vi "Set Double.vi"(8 "error in":errorcluster, 9 "value":dbl, 10 "variable name":string, 11 "GOLPI ref. in":T1={"pipe handle"={"lv_proc.dll file path"=path "", "process instance handle"=[]}, "fast read timeout [ms]"=500, "fast read settle time [ms]"=10, "fast read to multiple [ms]"=1, "max elements per input line"=100}) -> (0 "error out":errorcluster, 3 "GOLPI ref. out":T1={"pipe handle"={"lv_proc.dll file path"=path "", "process instance handle"=[]}, "fast read timeout [ms]"=500, "fast read settle time [ms]"=10, "fast read to multiple [ms]"=1, "max elements per input line"=100})   [LabVIEW 2013, in "GOLPI library.lvlib"]
uses:
  GOLPI library.lvlib
  Type Definitions/GOLPI reference Type Def.ctl
  LV Process.lvlibp/Pipe Handle.ctl
  LV Process.lvlibp
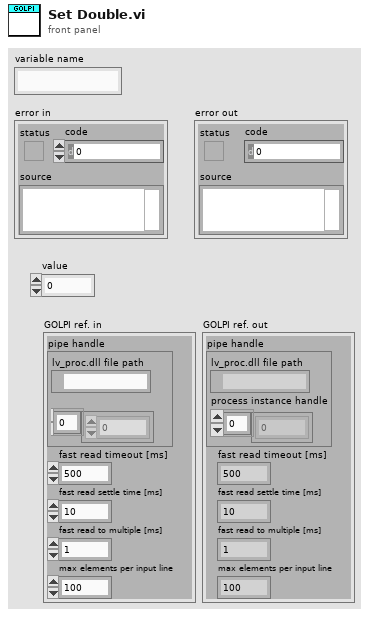
[diagram p1: front panel]
types:
  T1 = typedef "GOLPI library.lvlib/GOLPI reference Type Def.ctl" = cluster{"pipe handle":T2, "fast read timeout [ms]":u32, "fast read settle time [ms]":u32, "fast read to multiple [ms]":u32, "max elements per input line":u32}
  T2 = typedef "LV Process.lvlibp/Pipe Handle.ctl" = cluster{"lv_proc.dll file path":path, "process instance handle":u32[]}
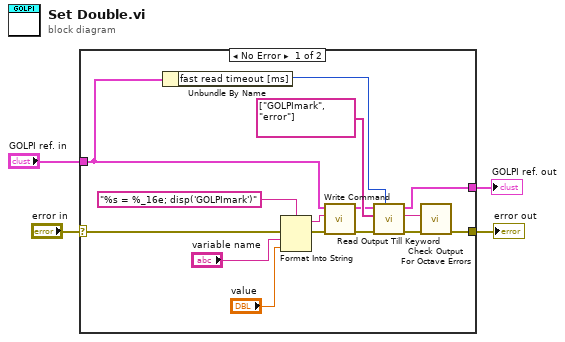
[diagram p0: block diagram]
diagram:
  n1 = case shown="No Error" "error in" {
    selector: "error in" -> [w16 w21]
    tunnel: [w8 w21] -> w4
    tunnel: "GOLPI ref. in" -> [w6 w20]
    tunnel: [w7 w20] -> w1
    frame No Error {
      n2 = Unbundle By Name(w6) -> ("fast read timeout [ms]"=w5:u32)
      n3 = Format Into String(format string="%s = %_16e; disp('GOLPImark')", error in=w16, "variable name", "value") -> (resulting string=w14:string, error out=w15:errorcluster)  [unwired: 1 in]
      n4 = call "Write Command.vi"("error in"=w15, "command"=w14, "GOLPI ref. in"=w6) -> ("error out"=w13:errorcluster, "GOLPI ref. out"=w10:T1)  [unwired: 7 in]
      n5 = call "Read Output Till Keyword.vi"("timeout [ms]"=w5, "error in"=w13, "keywords"=string[] ["GOLPImark", "error"], "GOLPI ref. in"=w10) -> ("error out"=w12:errorcluster, "read buffer"=w9:string, "GOLPI ref. out"=w7:T1)  [unwired: 4 in, 1 out]
      n6 = call "Check Output For Octave Errors.vi"("error in"=w12, "read buffer"=w9) -> ("error out"=w8:errorcluster)  [unwired: 9 in]
    }
    frame Error {
    }
  }
  "error out" <- w4
  "GOLPI ref. out" <- w1
